vi "AVI-Read.vi"() -> (0 "ErrOut":errorcluster)   [LabVIEW 2016]
doc: "Use this template to build a VI to use as a subVI."
panel:
  out "Image":T1(plugin-control)
  in  "ErrIn":errorcluster
  # "Input Parameters"
  # "Output Parameters"
  # "VI Description:\nThis VI is .."
  # ":: MVI Framework V1.0 ::\nAuthor:Gaoke Yang\nEmail: gaoke.yang@yahoo.com\nWeb: www.mvicontrol.com\nCopyright (C) 2014, MVI Technologies All Rights Reserved"
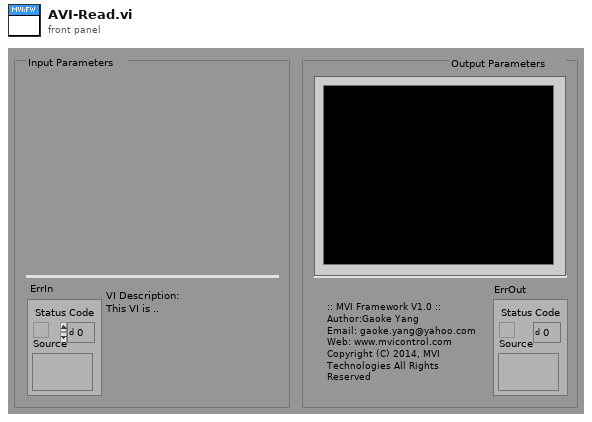
[diagram p1: front panel]
types:
  T1 = typedef "IMAQ Image.ctl" = refnum<image>
  T2 = typedef "IMAQ AVI2 Refnum.ctl" = refnum<k20>
  T3 = typedef "Image Type" = u32
  T4 = cluster{"Width":u32, "Height":u32, "Frames Per Second":u32, "Codec":string, "Has Data":bool}
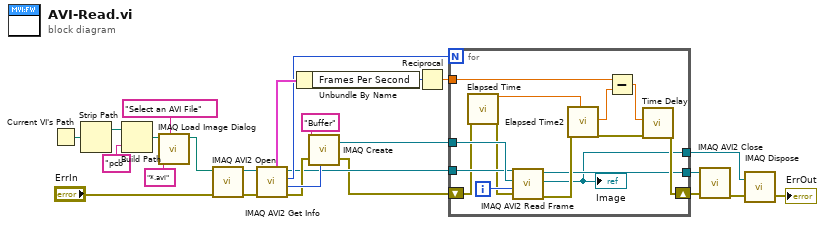
[diagram p0: block diagram]
diagram:
  n1 = Current VI's Path() -> (path=w21:path)
  n2 = Strip Path(path=w21) -> (stripped path=w20:path)  [unwired: 1 out]
  n3 = Build Path(base path=w20, name or relative path="pcb") -> (appended path=w14:path)
  n4 = call "IMAQ Load Image Dialog"("Prompt"="Select an AVI File" ("prompt"), "Pattern"="*.avi", "Start Path"=w14) -> ("Path"=w18:path)  [unwired: 6 in, 2 out]
  n5 = call "IMAQ AVI2 Open"("error in (no error)"="ErrIn", "AVI File Path"=w18) -> ("error out"=w15:errorcluster, "AVI Refnum"=w16:T2)  [unwired: 1 in, 7 out]
  n6 = call "IMAQ AVI2 Get Info"("error in (no error)"=w15, "AVI Refnum"=w16) -> ("error out"=w9:errorcluster, "Image Type"=w10:T3, "Number of Frames"=w6:u32, "AVI Refnum (duplicate)"=w5:T2, "Frame Data"=w12:T4)  [unwired: 5 out]
  n7 = Unbundle By Name(w12) -> ("Frames Per Second"=w7:u32)
  n8 = call "IMAQ Create"("Image Name"="Buffer", "Image Type"=w10, "error in (no error)"=w9) -> ("New Image"=w8:T1, "error out"=w4:errorcluster)  [unwired: 1 in, 1 out]
  n9 = Reciprocal(x=w7) -> (1/x=w3:dbl)
  n10 = for {
    N: w6 -> [_]
    shift-right: [w28] -> w24
    shift-left: w4 -> [w36]
    tunnel: w8 -> [w38]
    tunnel: w5 -> [w37]
    tunnel: w3 -> [w32]
    tunnel: [w27] -> w2
    tunnel: [w26] -> w1
    i -> [w39]
    n11 = call "Elapsed Time"("error in (no error)"=w36) -> ("Present (s)"=w34:dbl, "error out"=w35:errorcluster)  [unwired: 11 in, 6 out]
    n12 = call "IMAQ AVI2 Read Frame"("error in (no error)"=w35, "Frame Number"=w39, "Image"=w38, "AVI Refnum"=w37) -> ("error out"=w33:errorcluster, "Image Out"=w26:T1, "AVI Refnum (duplicate)"=w27:T2)  [unwired: 5 out]
    "Image" <- w26
    n13 = call "Elapsed Time2"("error in (no error)"=w33, "Set Start Time (s)"=w34) -> ("Elapsed Time (s)"=w31:dbl, "error out"=w29:errorcluster)  [unwired: 10 in, 6 out]
    n14 = Subtract(x=w32, y=w31) -> (x-y=w30:dbl)
    n15 = call "Time Delay"("error in (no error)"=w29, "Delay Time (s)"=w30) -> ("error out"=w28:errorcluster)  [unwired: 9 in]
  }
  n16 = call "IMAQ AVI2 Close"("error in (no error)"=w24, "AVI Refnum"=w2) -> ("error out"=w23:errorcluster)  [unwired: 9 in]
  n17 = call "IMAQ Dispose"("Image"=w1, "error in (no error)"=w23) -> ("error out"=→"ErrOut":errorcluster)  [unwired: 4 in]
